vi "SCM7 PS Control Remote3.vi"() -> ()   [LabVIEW 2025]
panel:
  in  "rate T":dbl format="%#_4g"
  in  "set T":dbl format="%#_4g"
  out "Tppms":dbl format="%#_4g"
  in  "Hold":bool
  out "error out 3":errorcluster={"status"=TRUE, "code"=1055, "source"="Close Reference in SCM PS Control Remote2.vi"}
  in  "menu":T1(ring)
  in  "Slew Rate [T/min]":dbl=0.2 format="%#_4g"
  in  "Setpoint [T]":dbl format="%#_4g"
  in  "stop":bool
  in  "port":u16=3375
  in  "error in (no error) 2":errorcluster
  in  "Data mac ip address":string="146.201.200.173"
  out "Field [T]":dbl format="%#_4g"
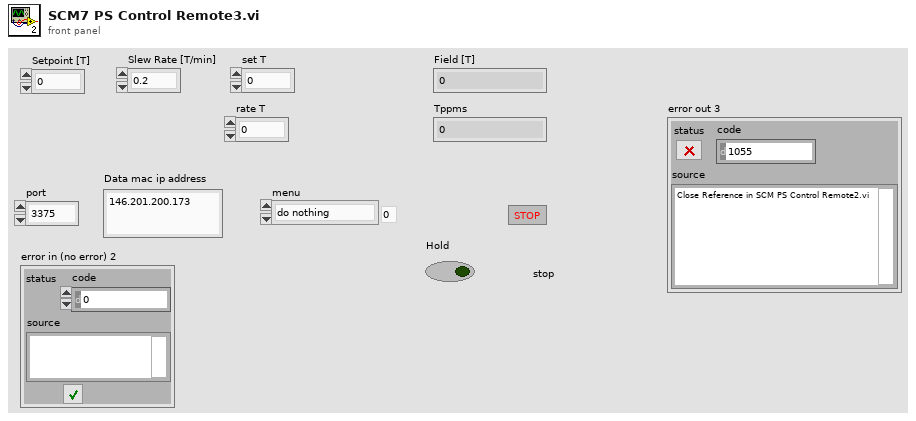
[diagram p1: front panel]
types:
  T1 = enum16{"do nothing", "Ramp To Setpoint", "change set point", "change slew rate", "change Tppms", "change rate T"}
  T2 = enum16{"do nothing", "Ramp To Setpoint", "change set point", "change slew rate"}
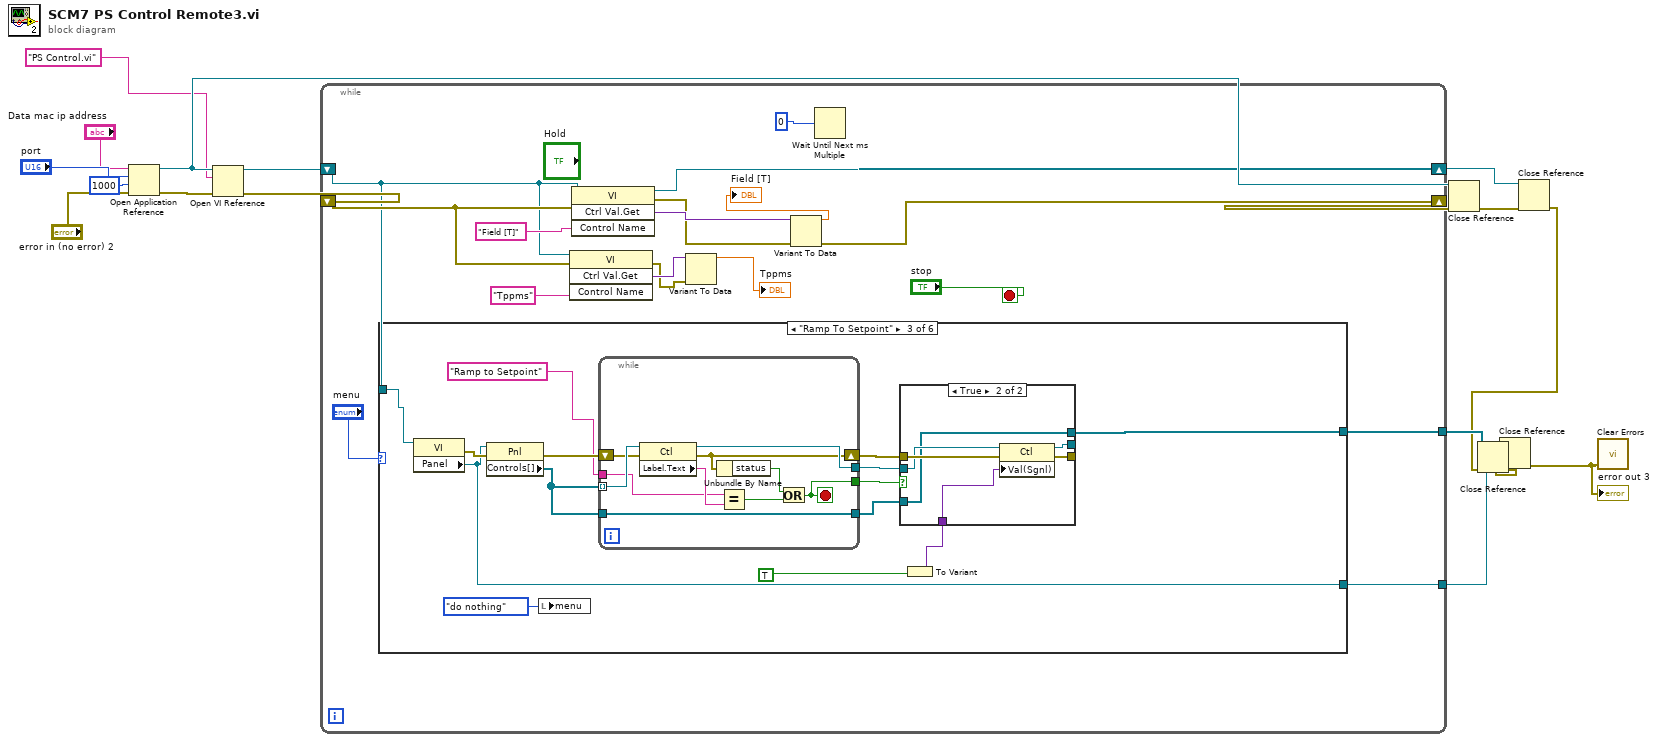
[diagram p0: block diagram]
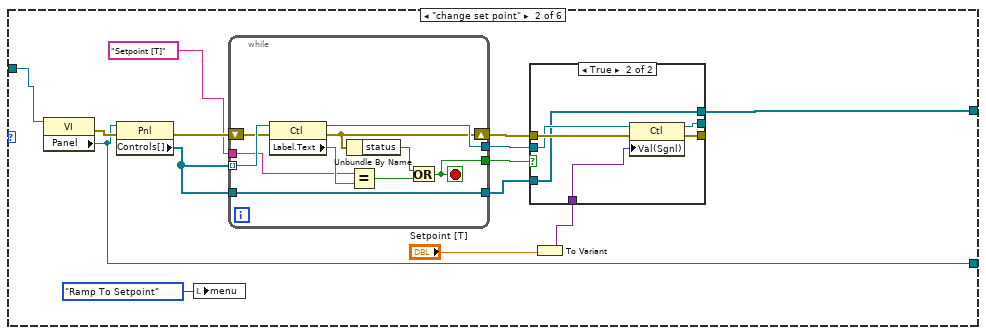
[diagram p3: hidden frame]
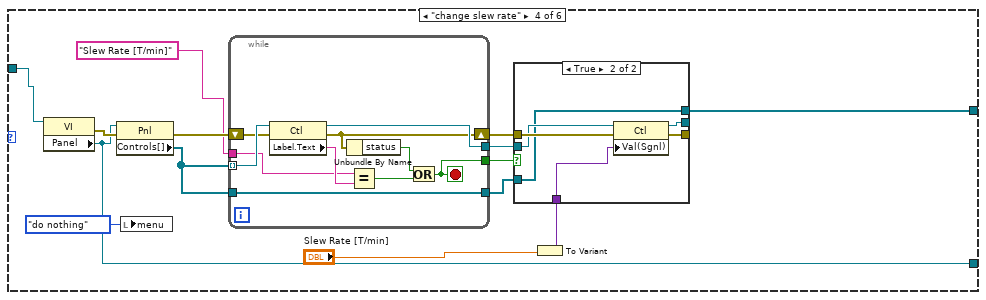
[diagram p6: hidden frame]
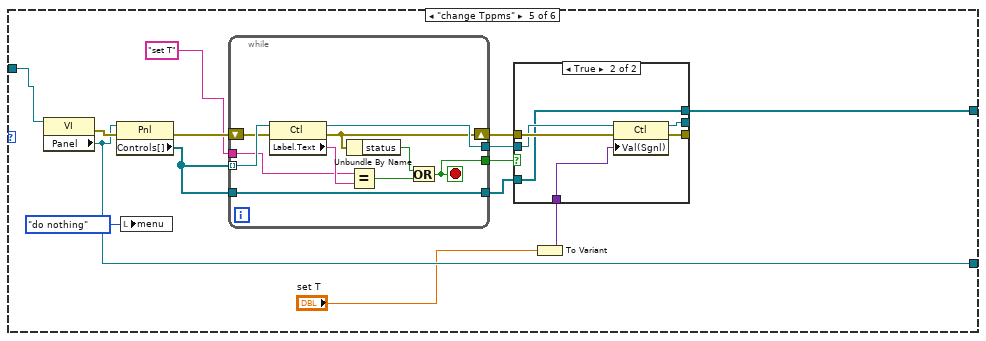
[diagram p8: hidden frame]
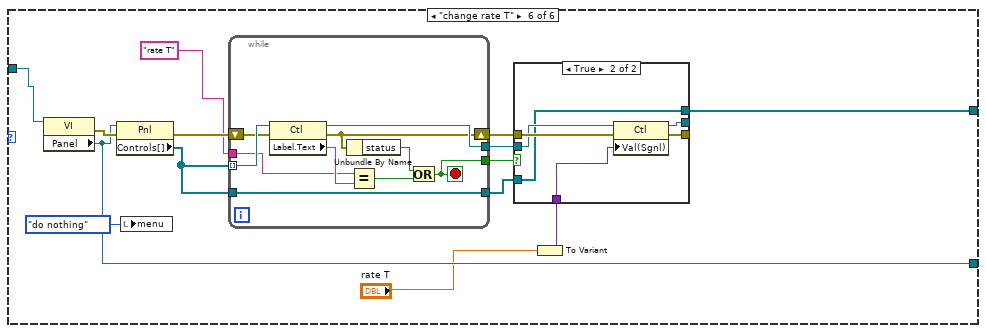
[diagram p10: hidden frame]
diagram:
  n1 = Open Application Reference(8:"error in (no error) 2", 9:1000 ("timeout ms (60000)"), 10:"port", 11:"Data mac ip address") -> (0:w16:errorcluster, 3:w10:refnum<vi>)
  n2 = Open VI Reference(application reference (local)=w10, vi path="PS Control.vi" ("VI name"), error in (no error)=w16) -> (vi reference=w8:refnum<vi>, error out=w13:errorcluster)  [unwired: 3 in]
  n3 = while {
    shift-right: [w32] -> w9
    shift-left: w8 -> [w21]
    shift-right: [w34] -> w12
    shift-left: w13 -> [w22]
    tunnel: [w25] -> w5
    tunnel: [w24] -> w4
    stop <- "stop" stop-if-true
    n4 = case shown="\"Ramp To Setpoint\"" "menu" {
      tunnel: w21 -> [_ w38 w72 w105 w138 w171]
      tunnel: [_ w37 w71 w103 w137 w170] -> w25
      tunnel: [_ w36 w70 w102 w136 w169] -> w24
      frame "do nothing", Default {
      }
      frame "change set point" {
        n5 = property class="VI"(reference=w38) -> (error out=w47:errorcluster, "Panel"=w36:refnum<vi>)  [unwired: 1 in, 1 out]
        n6 = property class="Pnl"(reference=w36, error in=w47) -> (error out=w46:errorcluster, "Controls[]"=w48:refnum<vi>[])  [unwired: 1 out]
        n7 = local write "menu"(T2."Ramp To Setpoint" ("menu")) -> ()
        n8 = while {
          tunnel: w48 -> [w67] mode=indexing
          tunnel: "Setpoint [T]" ("Control Name") -> [w65]
          shift-right: [w62] -> w43
          shift-left: w46 -> [w64]
          tunnel: [w63] -> w45
          tunnel: [w59] -> w44
          tunnel: w48 -> [w58]
          tunnel: [w58] -> w42
          stop <- w59 stop-if-true
          n9 = property class="Ctl"(reference=w67, error in=w64) -> (reference out=w63:refnum<vi>, error out=w62:errorcluster, "Label.Text"=w66:string)
          n10 = Unbundle By Name(w62) -> ("status"=w61:bool)
          n11 = Equal?(x=w65, y=w66) -> (x = y?=w60:bool)
          n12 = Or(x=w61, y=w60) -> (x .or. y?=w59:bool)
        }
        n13 = To Variant(anything="Setpoint [T]") -> (Variant=w40:variant)
        n14 = case shown="True" w44 {
          tunnel: w45 -> [w50 w56]
          tunnel: w43 -> [w51 w57]
          tunnel: [w51 w55] -> _
          tunnel: [w50 w54] -> _
          tunnel: w42 -> [w49 w53]
          tunnel: [w49 w53] -> w37
          tunnel: w40 -> [_ w52]
          frame False {
          }
          frame True {
            n15 = property class="Ctl"(reference=w56, error in=w57, "Val(Sgnl)"=w52) -> (reference out=w54:refnum<vi>, error out=w55:errorcluster)
          }
        }
      }
      frame "Ramp To Setpoint" {
        n16 = property class="VI"(reference=w72) -> (error out=w80:errorcluster, "Panel"=w70:refnum<vi>)  [unwired: 1 in, 1 out]
        n17 = property class="Pnl"(reference=w70, error in=w80) -> (error out=w79:errorcluster, "Controls[]"=w81:refnum<vi>[])  [unwired: 1 out]
        n18 = local write "menu"(T2."do nothing" ("menu")) -> ()
        n19 = while {
          tunnel: w81 -> [w100] mode=indexing
          tunnel: "Ramp to Setpoint" ("Control Name") -> [w98]
          shift-right: [w95] -> w76
          shift-left: w79 -> [w97]
          tunnel: [w96] -> w78
          tunnel: [w92] -> w77
          tunnel: w81 -> [w91]
          tunnel: [w91] -> w75
          stop <- w92 stop-if-true
          n20 = property class="Ctl"(reference=w100, error in=w97) -> (reference out=w96:refnum<vi>, error out=w95:errorcluster, "Label.Text"=w99:string)
          n21 = Unbundle By Name(w95) -> ("status"=w94:bool)
          n22 = Equal?(x=w98, y=w99) -> (x = y?=w93:bool)
          n23 = Or(x=w94, y=w93) -> (x .or. y?=w92:bool)
        }
        n24 = To Variant(anything=TRUE) -> (Variant=w73:variant)
        n25 = case shown="True" w77 {
          tunnel: w78 -> [w83 w89]
          tunnel: w76 -> [w84 w90]
          tunnel: [w84 w88] -> _
          tunnel: [w83 w87] -> _
          tunnel: w75 -> [w82 w86]
          tunnel: [w82 w86] -> w71
          tunnel: w73 -> [_ w85]
          frame False {
          }
          frame True {
            n26 = property class="Ctl"(reference=w89, error in=w90, "Val(Sgnl)"=w85) -> (reference out=w87:refnum<vi>, error out=w88:errorcluster)
          }
        }
      }
      frame "change slew rate" {
        n27 = property class="VI"(reference=w105) -> (error out=w113:errorcluster, "Panel"=w102:refnum<vi>)  [unwired: 1 in, 1 out]
        n28 = property class="Pnl"(reference=w102, error in=w113) -> (error out=w112:errorcluster, "Controls[]"=w114:refnum<vi>[])  [unwired: 1 out]
        n29 = local write "menu"(T2."do nothing" ("menu")) -> ()
        n30 = while {
          tunnel: w114 -> [w133] mode=indexing
          tunnel: "Slew Rate [T/min]" ("Control Name") -> [w131]
          shift-right: [w128] -> w109
          shift-left: w112 -> [w130]
          tunnel: [w129] -> w111
          tunnel: [w125] -> w110
          tunnel: w114 -> [w124]
          tunnel: [w124] -> w108
          stop <- w125 stop-if-true
          n31 = property class="Ctl"(reference=w133, error in=w130) -> (reference out=w129:refnum<vi>, error out=w128:errorcluster, "Label.Text"=w132:string)
          n32 = Unbundle By Name(w128) -> ("status"=w127:bool)
          n33 = Equal?(x=w131, y=w132) -> (x = y?=w126:bool)
          n34 = Or(x=w127, y=w126) -> (x .or. y?=w125:bool)
        }
        n35 = To Variant(anything="Slew Rate [T/min]") -> (Variant=w106:variant)
        n36 = case shown="True" w110 {
          tunnel: w111 -> [w116 w122]
          tunnel: w109 -> [w117 w123]
          tunnel: [w117 w121] -> _
          tunnel: [w116 w120] -> _
          tunnel: w108 -> [w115 w119]
          tunnel: [w115 w119] -> w103
          tunnel: w106 -> [_ w118]
          frame False {
          }
          frame True {
            n37 = property class="Ctl"(reference=w122, error in=w123, "Val(Sgnl)"=w118) -> (reference out=w120:refnum<vi>, error out=w121:errorcluster)
          }
        }
      }
      frame "change Tppms" {
        n38 = property class="VI"(reference=w138) -> (error out=w146:errorcluster, "Panel"=w136:refnum<vi>)  [unwired: 1 in, 1 out]
        n39 = property class="Pnl"(reference=w136, error in=w146) -> (error out=w145:errorcluster, "Controls[]"=w147:refnum<vi>[])  [unwired: 1 out]
        n40 = local write "menu"(T2."do nothing" ("menu")) -> ()
        n41 = while {
          tunnel: w147 -> [w166] mode=indexing
          tunnel: "set T" ("Control Name") -> [w164]
          shift-right: [w161] -> w142
          shift-left: w145 -> [w163]
          tunnel: [w162] -> w144
          tunnel: [w158] -> w143
          tunnel: w147 -> [w157]
          tunnel: [w157] -> w141
          stop <- w158 stop-if-true
          n42 = property class="Ctl"(reference=w166, error in=w163) -> (reference out=w162:refnum<vi>, error out=w161:errorcluster, "Label.Text"=w165:string)
          n43 = Unbundle By Name(w161) -> ("status"=w160:bool)
          n44 = Equal?(x=w164, y=w165) -> (x = y?=w159:bool)
          n45 = Or(x=w160, y=w159) -> (x .or. y?=w158:bool)
        }
        n46 = To Variant(anything="set T") -> (Variant=w139:variant)
        n47 = case shown="True" w143 {
          tunnel: w144 -> [w149 w155]
          tunnel: w142 -> [w150 w156]
          tunnel: [w150 w154] -> _
          tunnel: [w149 w153] -> _
          tunnel: w141 -> [w148 w152]
          tunnel: [w148 w152] -> w137
          tunnel: w139 -> [_ w151]
          frame False {
          }
          frame True {
            n48 = property class="Ctl"(reference=w155, error in=w156, "Val(Sgnl)"=w151) -> (reference out=w153:refnum<vi>, error out=w154:errorcluster)
          }
        }
      }
      frame "change rate T" {
        n49 = property class="VI"(reference=w171) -> (error out=w179:errorcluster, "Panel"=w169:refnum<vi>)  [unwired: 1 in, 1 out]
        n50 = property class="Pnl"(reference=w169, error in=w179) -> (error out=w178:errorcluster, "Controls[]"=w180:refnum<vi>[])  [unwired: 1 out]
        n51 = local write "menu"(T2."do nothing" ("menu")) -> ()
        n52 = while {
          tunnel: w180 -> [w199] mode=indexing
          tunnel: "rate T" ("Control Name") -> [w197]
          shift-right: [w194] -> w175
          shift-left: w178 -> [w196]
          tunnel: [w195] -> w177
          tunnel: [w191] -> w176
          tunnel: w180 -> [w190]
          tunnel: [w190] -> w174
          stop <- w191 stop-if-true
          n53 = property class="Ctl"(reference=w199, error in=w196) -> (reference out=w195:refnum<vi>, error out=w194:errorcluster, "Label.Text"=w198:string)
          n54 = Unbundle By Name(w194) -> ("status"=w193:bool)
          n55 = Equal?(x=w197, y=w198) -> (x = y?=w192:bool)
          n56 = Or(x=w193, y=w192) -> (x .or. y?=w191:bool)
        }
        n57 = To Variant(anything="rate T") -> (Variant=w172:variant)
        n58 = case shown="True" w176 {
          tunnel: w177 -> [w182 w188]
          tunnel: w175 -> [w183 w189]
          tunnel: [w183 w187] -> _
          tunnel: [w182 w186] -> _
          tunnel: w174 -> [w181 w185]
          tunnel: [w181 w185] -> w170
          tunnel: w172 -> [_ w184]
          frame False {
          }
          frame True {
            n59 = property class="Ctl"(reference=w188, error in=w189, "Val(Sgnl)"=w184) -> (reference out=w186:refnum<vi>, error out=w187:errorcluster)
          }
        }
      }
    }
    n60 = invoke class="VI" method="Ctrl Val.Get"(reference=w21, error in=w22, "Control Name"="Tppms") -> (error out=w19:errorcluster, "Get Control Value Variant"=w20:variant)  [unwired: 1 in, 2 out]
    n61 = invoke class="VI" method="Ctrl Val.Get"(reference=w21, error in=w22, "Control Name"="Field [T]") -> (reference out=w32:refnum<vi>, error out=w30:errorcluster, "Get Control Value Variant"=w31:variant)  [unwired: 1 in, 1 out]
    n62 = Variant To Data(error in=w19, Variant=w20) -> (data=→"Tppms":dbl)  [unwired: 1 in, 1 out]
    n63 = Variant To Data(error in=w30, Variant=w31) -> (data=→"Field [T]":dbl, error out=w34:errorcluster)  [unwired: 1 in]
    n64 = Wait Until Next ms Multiple(millisecond multiple=u32 0) -> ()  [unwired: 1 out]
  }
  n65 = Close Reference(reference=w10, error in (no error)=w12) -> (error out=w11:errorcluster)
  n66 = Close Reference(reference=w9, error in (no error)=w11) -> (error out=w2:errorcluster)
  n67 = Close Reference(reference=w5, error in (no error)=w2) -> (error out=w6:errorcluster)
  n68 = Close Reference(reference=w4, error in (no error)=w6) -> (error out=w3:errorcluster)
  "error out 3" <- w3
  n69 = call <vilib>:"Clear Errors.vi"("error in (no error)"=w3) -> ()  [unwired: 5 in, 2 out]
